vi "Write to TDMS.vi"(8 "error in (no error)":errorcluster, 10 "TDMS File Ref":refnum<k34>, 11 "1D Waveform Logging Data in":refnum<class "1D Waveform Logging Data.lvclass">) -> (0 "error out":errorcluster)   [LabVIEW 2024, in "Logging Data.lvlib" / "1D Waveform Logging Data.lvclass"]
uses:
  1D Waveform Logging Data.lvclass
  C:/Users/uspoaotto/OneDrive - Oregon Tool/Desktop/working copies/dataLogger/Logging Data/Logging Data/Logging Data.lvclass
  1D Waveform Logging Data.lvclass/1D Waveform Logging Data.ctl
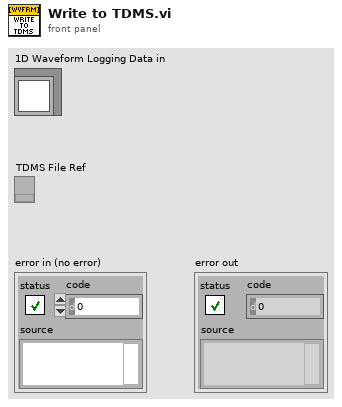
[diagram p1: front panel]
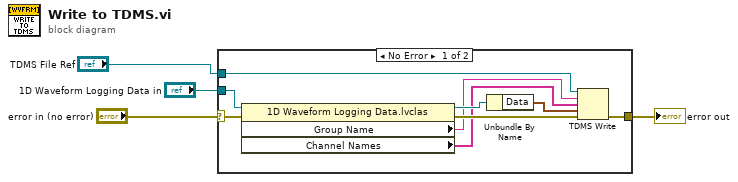
[diagram p0: block diagram]
diagram:
  n1 = case shown="No Error" "error in (no error)" {
    selector: "error in (no error)" -> [w10 w14]
    tunnel: "1D Waveform Logging Data in" -> [w12 _]
    tunnel: "TDMS File Ref" -> [w6 _]
    tunnel: [w5 w14] -> w1
    frame No Error {
      n2 = property class="1D Waveform Logging Data.lvclas"(reference=w12, error in=w10) -> (reference out=w11:refnum<class "1D Waveform Logging Data.lvclass">, error out=w9:errorcluster, "Group Name"=w8:string, "Channel Names"=w7:string[])
      n3 = Unbundle By Name(w11) -> ("Data"=w13:waveform(dbl)[])
      n4 = TDMS Write(0:w6, 5:w8, 7:w7, 9:w13, 11:w9) -> (15:w5:errorcluster)  [unwired: 1 in, 3 out]
    }
    frame Error {
    }
  }
  "error out" <- w1
